vi "GlobalMeasure.vi"() -> ()   [LabVIEW 2014]
panel:
  in  "MeasureResultRP":T1 {"ZBRPCCWAImF" format="%.2f"; "ZBRPCCWAvgF" format="%.2f"; "ZBRPCCWVarF" format="%.2f"; "ZBRPCCWLoF" format="%.2f"; "ZBRPCCWHiF" format="%.2f"; "ZBRPCWAvgF" format="%.2f"; "ZBRPCWVarF" format="%.2f"; "ZBRPCWLoF" format="%.2f"; "ZBRPCWHiF" format="%.2f"; "ZARPCCWAImF" format="%.2f"; "ZARPCCWAvgF" format="%.2f"; "ZARPCCWVarF" format="%.2f"; "ZARPCCWLoF" format="%.2f"; "ZARPCCWHiF" format="%.2f"; "ZARPCWAvgF" format="%.2f"; "ZARPCWVarF" format="%.2f"; "ZARPCWLoF" format="%.2f"; "ZARPCWHiF" format="%.2f"}
  in  "MeasureResultPT":T2 {"ZBPTCCWAImT" format="%.2f"; "ZBPTCCWAvgT" format="%.2f"; "ZBPTCCWVarT" format="%.2f"; "ZBPTCCWLoT" format="%.2f"; "ZBPTCCWHiT" format="%.2f"; "ZBPTCWAvgT" format="%.2f"; "ZBPTCWVarT" format="%.2f"; "ZBPTCWLoT" format="%.2f"; "ZBPTCWHiT" format="%.2f"; "ZAPTCCWAImT" format="%.2f"; "ZAPTCCWAvgT" format="%.2f"; "ZAPTCCWVarT" format="%.2f"; "ZAPTCCWLoT" format="%.2f"; "ZAPTCCWHiT" format="%.2f"; "ZAPTCWAvgT" format="%.2f"; "ZAPTCWVarT" format="%.2f"; "ZAPTCWLoT" format="%.2f"; "ZAPTCWHiT" format="%.2f"}
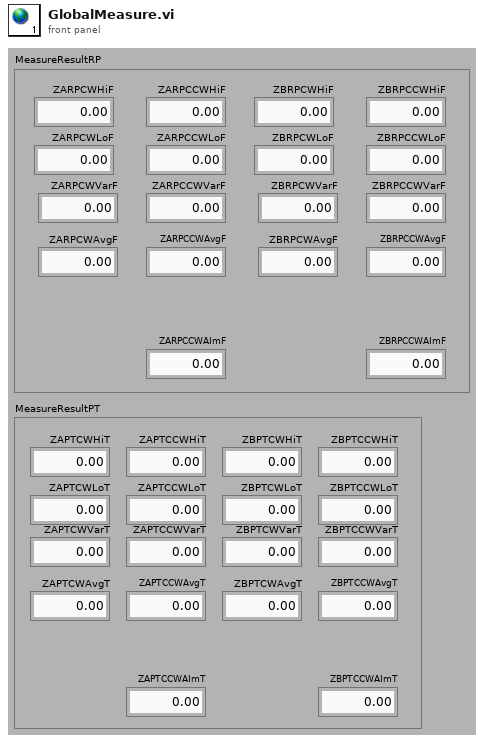
[diagram p1: front panel]
types:
  T1 = cluster{"ZARPCWHiF":sgl, "ZARPCWLoF":sgl, "ZARPCWVarF":sgl, "ZARPCWAvgF":sgl, "ZARPCCWHiF":sgl, "ZARPCCWLoF":sgl, "ZARPCCWVarF":sgl, "ZARPCCWAvgF":sgl, "ZARPCCWAImF":sgl, "ZBRPCWHiF":sgl, "ZBRPCWLoF":sgl, "ZBRPCWVarF":sgl, "ZBRPCWAvgF":sgl, "ZBRPCCWHiF":sgl, "ZBRPCCWLoF":sgl, "ZBRPCCWVarF":sgl, "ZBRPCCWAvgF":sgl, "ZBRPCCWAImF":sgl}
  T2 = cluster{"ZAPTCWHiT":sgl, "ZAPTCWLoT":sgl, "ZAPTCWVarT":sgl, "ZAPTCWAvgT":sgl, "ZAPTCCWHiT":sgl, "ZAPTCCWLoT":sgl, "ZAPTCCWVarT":sgl, "ZAPTCCWAvgT":sgl, "ZAPTCCWAImT":sgl, "ZBPTCWHiT":sgl, "ZBPTCWLoT":sgl, "ZBPTCWVarT":sgl, "ZBPTCWAvgT":sgl, "ZBPTCCWHiT":sgl, "ZBPTCCWLoT":sgl, "ZBPTCCWVarT":sgl, "ZBPTCCWAvgT":sgl, "ZBPTCCWAImT":sgl}
diagram:
